vi "Select multiplexer LR700.vi"(8 "error in":errorcluster, 10 "Sensor <01-99>":i32=1 min=1 max=99, 11 "VISA Resource Name":refnum<visa-resource-name>) -> (0 "error out":errorcluster, 3 "VISA Resource Name Out":refnum<visa-resource-name>)   [LabVIEW 2015]
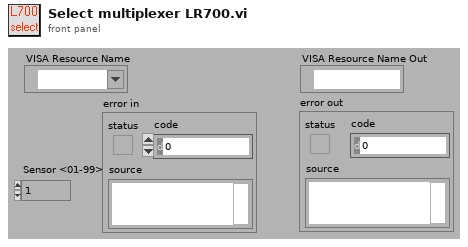
[diagram p1: front panel]
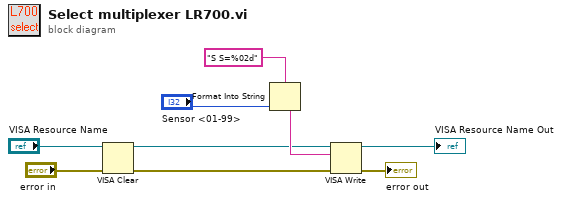
[diagram p0: block diagram]
diagram:
  n1 = VISA Clear(VISA resource name="VISA Resource Name", error in (no error)="error in") -> (VISA resource name out=w2:refnum<visa-resource-name>, error out=w4:errorcluster)
  n2 = Format Into String(format string="S S=%02d", "Sensor <01-99>") -> (resulting string=w7:string)  [unwired: 2 in, 1 out]
  n3 = VISA Write(VISA resource name=w2, write buffer=w7, error in (no error)=w4) -> (VISA resource name out=→"VISA Resource Name Out":refnum<visa-resource-name>, error out=→"error out":errorcluster)  [unwired: 1 out]
